vi "Reset Timing Statistics.vi"(8 "error in (no error)":errorcluster, 11 "ResultTree in":refnum<class "ResultTree.lvclass">) -> (0 "error out":errorcluster, 3 "ResultTree out":refnum<class "ResultTree.lvclass">)   [LabVIEW 2017, in "ResultTree.lvclass"]
uses:
  ResultTree.lvclass
  ResultTree.lvclass/ResultTree.ctl
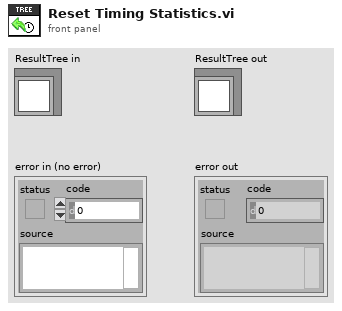
[diagram p1: front panel]
types:
  T1 = cluster{"Qualified Name":string, "Duration":dbl}[]
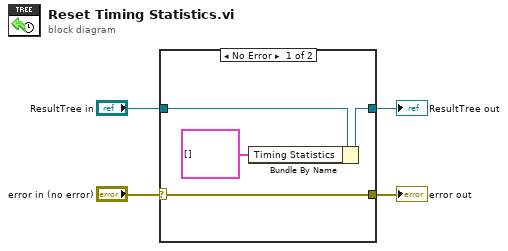
[diagram p0: block diagram]
diagram:
  n1 = case shown="No Error" "error in (no error)" {
    selector: "error in (no error)" -> [w7 w10]
    tunnel: [w7 w10] -> w3
    tunnel: [w6 w9] -> w1
    tunnel: "ResultTree in" -> [w8 w9]
    frame No Error {
      n2 = Bundle By Name(cluster=w8, "Timing Statistics"=T1 []) -> (w6:refnum<class "ResultTree.lvclass">)
    }
    frame Error {
    }
  }
  "error out" <- w3
  "ResultTree out" <- w1
